vi "Run Client.vi"(8 "error in":errorcluster, 10 "pin map context":T1, 11 "measurement configuration":T3) -> (0 "error out":errorcluster, 3 "measurement results":T2)   [LabVIEW 2021, in "Measurement Client Template.lvlib"]
doc: "<B>Run Client.vi</B> is a wrapper to demonstrate the working of Measurement Plug-In Client. It performs the following functions:\n\n- Create a client for the measurement service.\n- Run the measurement logic and display the results.\n - Start the measurement for the given measurement configuration.\n - Read and display the measurement results, until the measurement fails.\n - Stop the measurement.\n- Close the client connection.\n- Optional: Cancel ongoing measure call."
uses:
  Measurement Client Template.lvlib
  controls/Measurement Configuration.ctl
  controls/Measurement Results.ctl
  <vilib>/gRPC/Generated APIs/ni/measurementlink/measurement/v2/Measurement Service Client V2/RPC Messages/ni_measurementlink_PinMapContext.ctl
  <vilib>/gRPC/Generated APIs/ni/measurementlink/measurement/v2/Measurement Service Client V2/Measurement Service Client V2.lvlib
panel:
  in  "stop client":bool
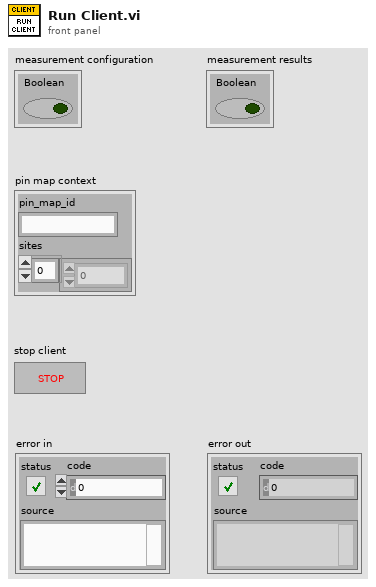
[diagram p1: front panel]
types:
  T1 = typedef "Measurement Service Client V2.lvlib/ni_measurementlink_PinMapContext.ctl" = cluster{"pin_map_id":string, "sites":i32[]}
  T2 = typedef "Measurement Client Template.lvlib/Measurement Results.ctl" = cluster{"Boolean":bool}
  T3 = typedef "Measurement Client Template.lvlib/Measurement Configuration.ctl" = cluster{"Boolean":bool}
  T4 = typedef "grpc-lvsupport-release.lvlib/grpcId.ctl" = u64
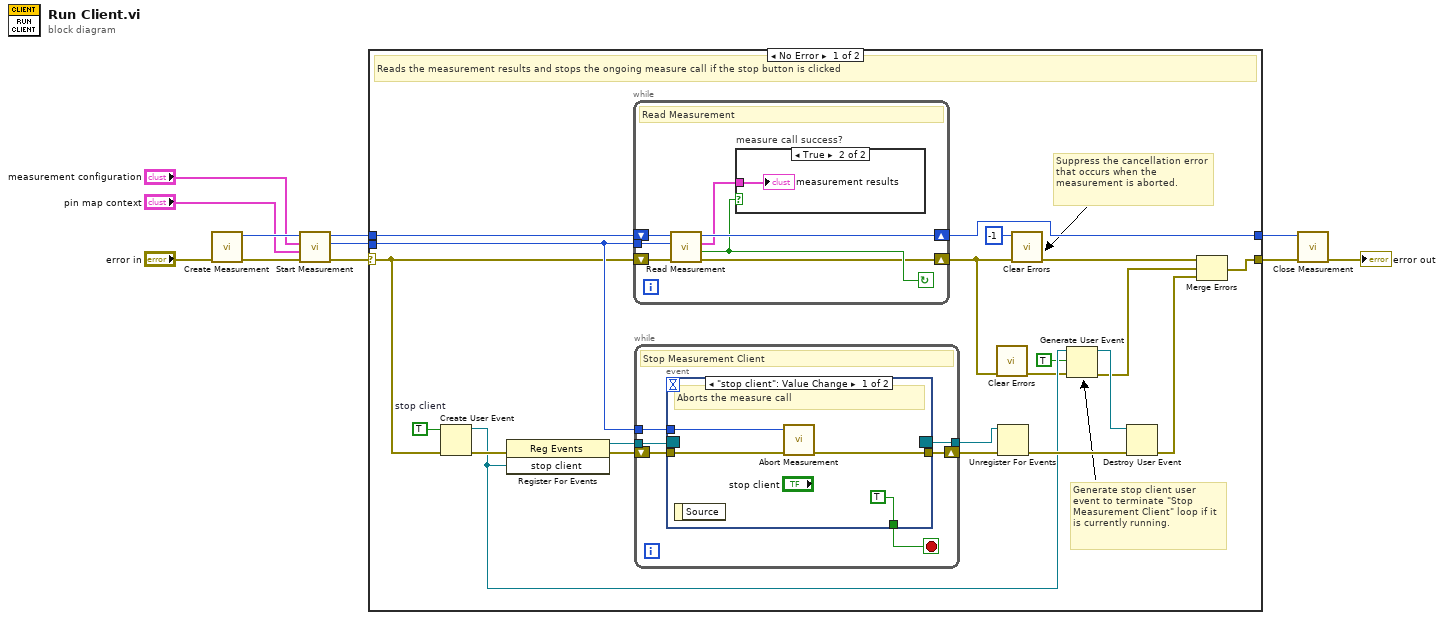
[diagram p0: block diagram]
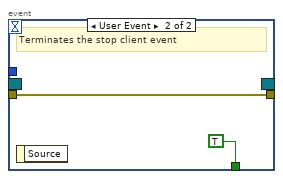
[diagram p2: hidden frame]
diagram:
  n1 = call "Create Measurement.vi"("error in"="error in") -> ("error out"=w11:errorcluster, "gRPCid out"=w9:T4)  [unwired: 9 in]
  n2 = call "Start Measurement.vi"("error in"=w11, "pin map context"="pin map context", "measurement configuration"="measurement configuration", "gRPCid in"=w9) -> ("error out"=w10:errorcluster, "call id"=w2:T4, "gRPCid out"=w6:T4)  [unwired: 5 in]
  n3 = case shown="No Error" w10 {
    selector: w10 -> [w19 w54]
    tunnel: w6 -> [w32 _]
    tunnel: [w13 w53] -> w4
    tunnel: w2 -> [w24 w53]
    tunnel: [w12 w54] -> w1
    frame No Error {
      w31 = TRUE  # stop client
      # "Suppress the cancellation error that occurs when the measurement is aborted."
      # "Generate stop client user event to terminate \"Stop Measurement Client\" loop if it is currently running."
      # "Reads the measurement results and stops the ongoing measure call if the stop button is clicked"
      n4 = Create User Event(user event datatype=w31, error in=w19) -> (user event=w22:refnum<user-event>, error out=w30:errorcluster)
      n5 = register-events(error in=w30, w22) -> (reference out=w29:refnum<event-registration>, error out=w28:errorcluster)  [unwired: 1 in]
      n6 = while {
        tunnel: w24 -> [w49]
        shift-right: [w45] -> w16
        shift-left: w19 -> [w51]
        shift-right: [w48] -> w13
        shift-left: w32 -> [w50]
        stop <- w46 continue-if-true
        # "Read Measurement"
        n7 = call "Read Measurement.vi"("error in"=w51, "call id"=w49, "gRPCid in"=w50) -> ("error out"=w45:errorcluster, "measure success?"=w46:bool, "measurement results"=w47:T2, "gRPCid out"=w48:T4)  [unwired: 5 in]
        n8 = case "measure call success?" shown="True" w46 {
          tunnel: w47 -> [_ w52]
          frame False {
          }
          frame True {
            "measurement results" <- w52
          }
        }
      }
      n9 = while {
        tunnel: w29 -> [w38]
        tunnel: [w37] -> w25
        shift-right: [w36] -> w27
        shift-left: w28 -> [w35]
        tunnel: w24 -> [w33]
        stop <- w34 stop-if-true
        # "Stop Measurement Client"
        n10 = event shown="[0] \"stop client\": Value Change" {
          selector: w38 -> [_ _]
          dyn-events: [_ _] -> w37
          timeout: _ -> [_ _]
          tunnel: w35 -> [w41 w44]
          tunnel: [w40 w44] -> w36
          tunnel: [TRUE TRUE] -> w34
          tunnel: w33 -> [w39 _]
          event "stop client": Value Change {
            # "Aborts the measure call"
            n11 = event-data() -> ()  [unwired: 1 in, 1 out]
            n12 = call "Abort Measurement.vi"("error in"=w41, "call ID in"=w39) -> ("error out"=w40:errorcluster)  [unwired: 9 in]
          }
          event User Event {
            # "Terminates the stop client event"
            n13 = event-data() -> ()  [unwired: 1 in, 1 out]
          }
        }
      }
      n14 = call <vilib>:"Clear Errors.vi"("error in (no error)"=w16) -> ("error out"=w21:errorcluster)  [unwired: 5 in, 1 out]
      n15 = Unregister For Events(event registration refnum=w25, error in=w27) -> (error out=w26:errorcluster)
      n16 = call <vilib>:"Clear Errors.vi"("error in (no error)"=w16, "specific error code to clear (0: all)"=-1) -> ("error out"=w15:errorcluster)  [unwired: 4 in, 1 out]
      n17 = Generate User Event(user event=w22, event data cluster=TRUE, error in=w21) -> (user event out=w23:refnum<user-event>, error out=w17:errorcluster)  [unwired: 1 in]
      n18 = Destroy User Event(user event=w23, error in=w26) -> (error out=w18:errorcluster)
      n19 = Merge Errors(w15, w17, w18) -> (w12:errorcluster)
    }
    frame Error {
      # "Pass"
    }
  }
  n20 = call "Close Measurement.vi"("error in"=w1, "gRPCid in"=w4) -> ("error out"=→"error out":errorcluster)  [unwired: 9 in]
